vi "add to cycle cluster.vi"(6 "data requested":string[](array[string])=["q", "ratio", "norm", "error", "percent error", "delta q", "use", "break"], 7 "charge state":dbl=3.0, 8 "error in":errorcluster, 11 "input cluster":T1 {"cycle results dbl" format="%#_11f"}) -> (0 "error out":errorcluster, 3 "output cluster":T1 {"cycle results dbl" format="%#_11f"})   [LabVIEW 2016]
uses:
  controls/cycle results control.ctl
panel:
  out "cycle results dbl 2":dbl[](array[numeric])
  out "cycle results labels 3":string[](array[string])
  out "appended array":dbl[][](array[numeric]) format="%#_6f"
  out "Array":dbl[][](array[numeric])
  out "cycle results labels 2":string[](array[string])
  out "cycle results dbl":dbl[][](array[numeric])
  out "cycle results labels":string[](array[string])
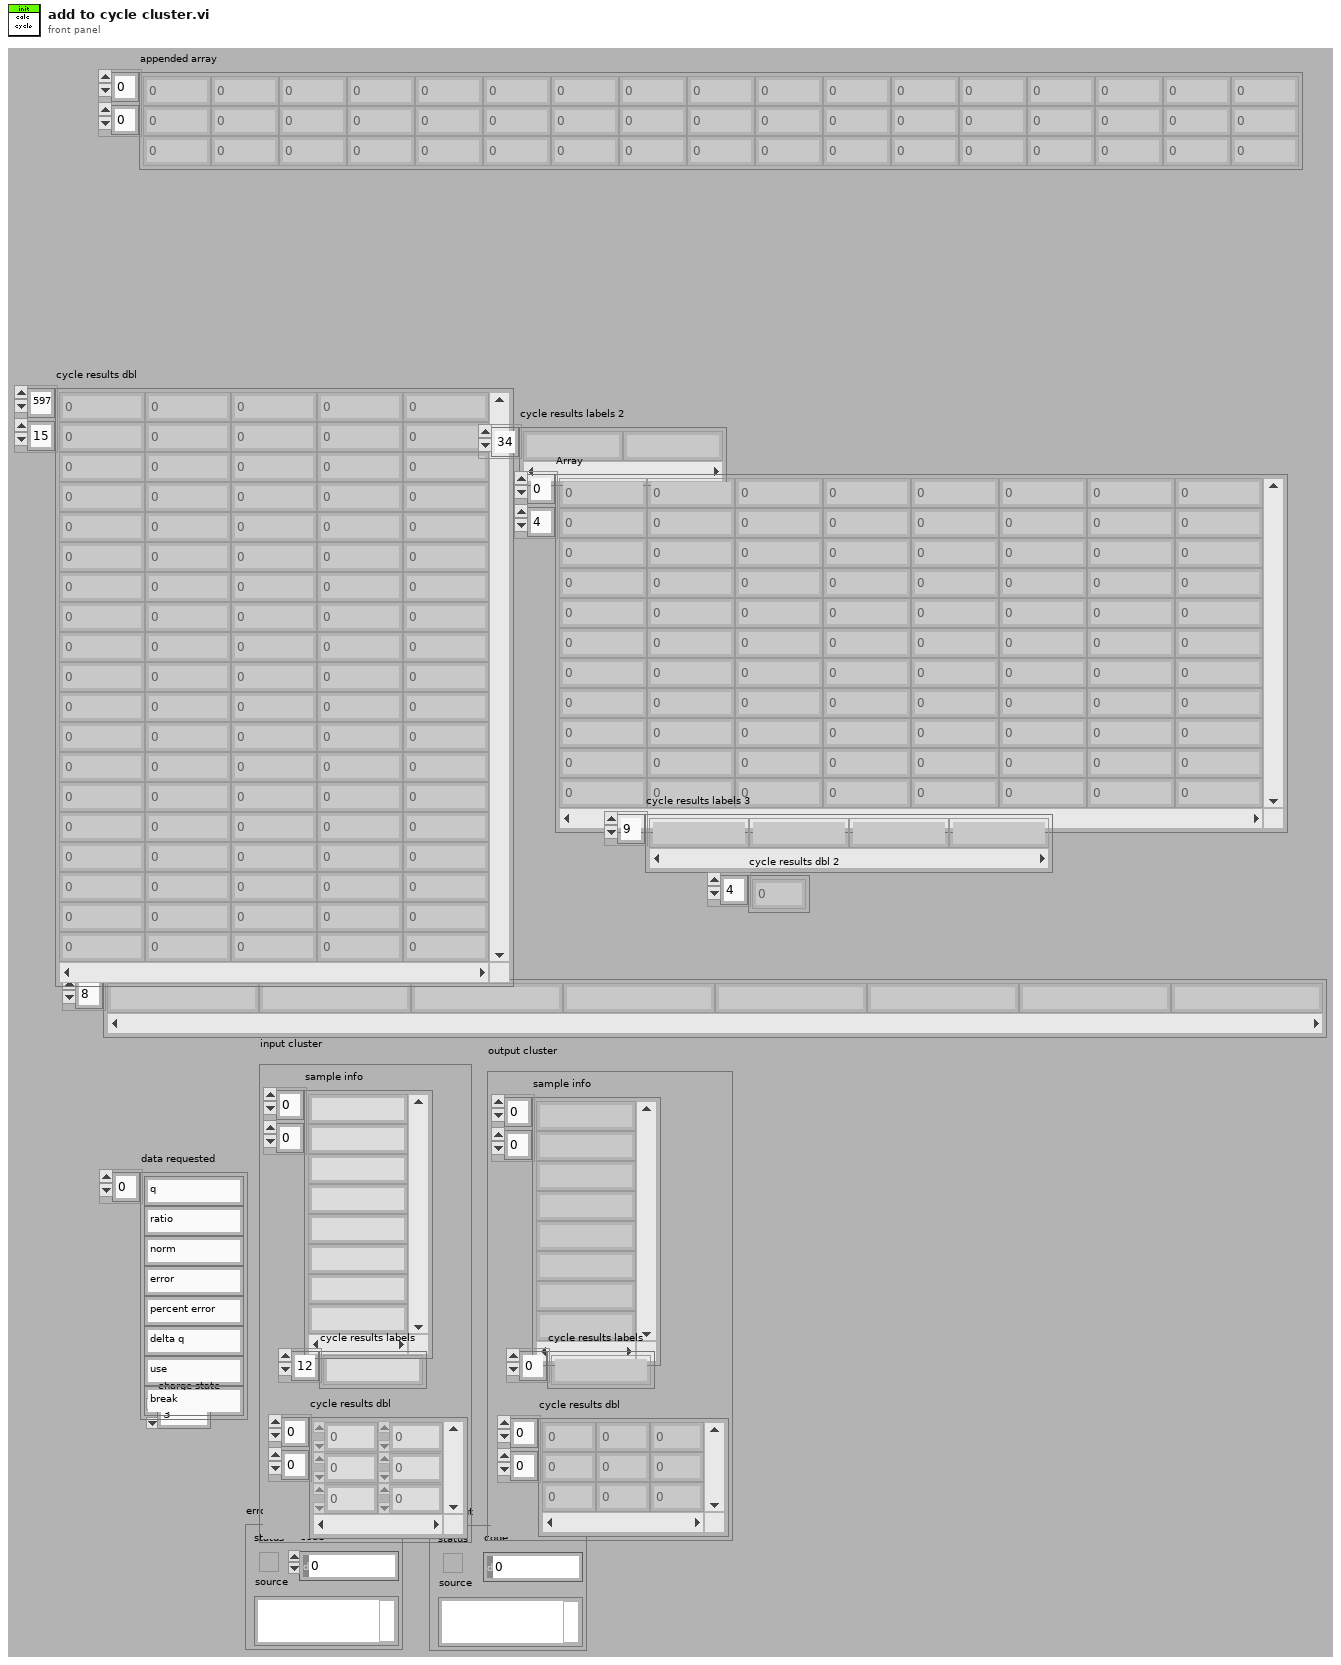
[diagram p1: front panel]
types:
  T1 = typedef "cycle results control.ctl" = cluster{"sample info":string[][], "cycle results labels":string[], "cycle results dbl":dbl[][]}
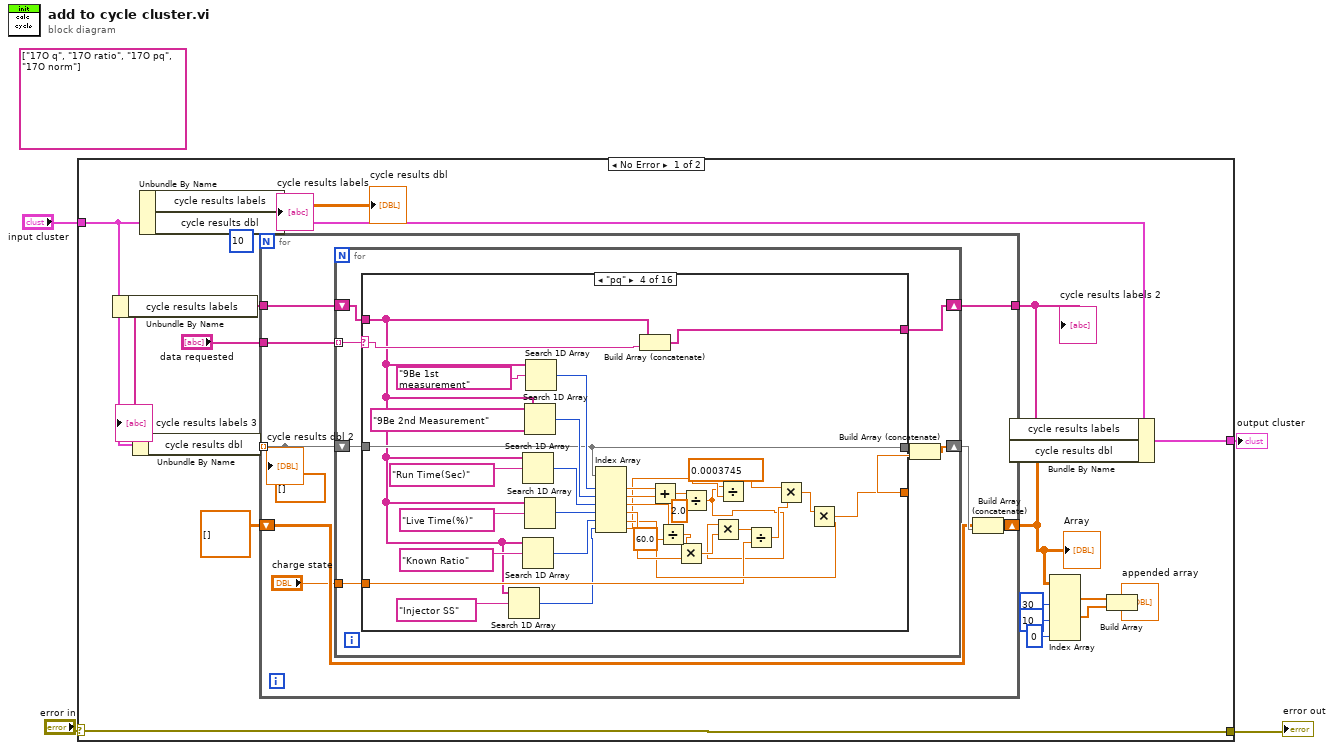
[diagram p0: block diagram]
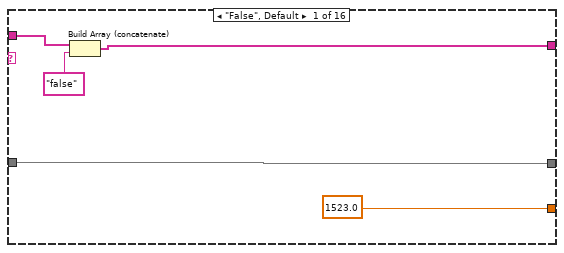
[diagram p2: hidden frame]
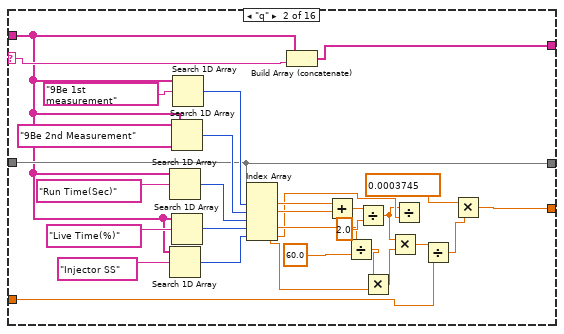
[diagram p3: hidden frame]
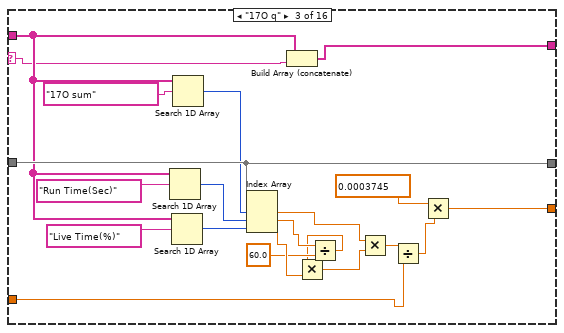
[diagram p4: hidden frame]
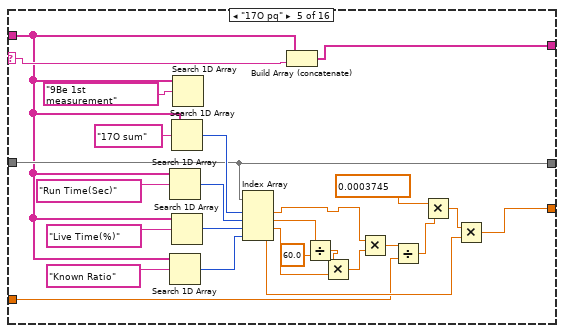
[diagram p5: hidden frame]
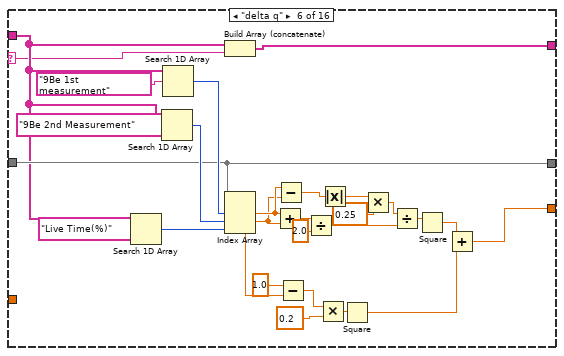
[diagram p6: hidden frame]
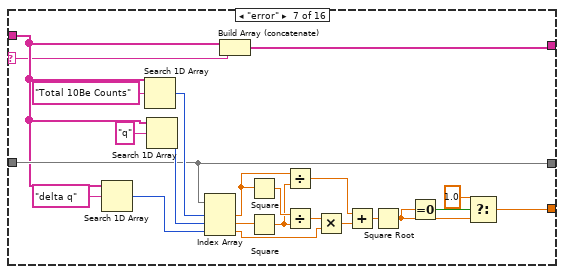
[diagram p7: hidden frame]
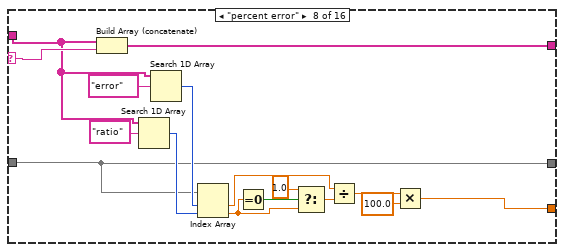
[diagram p8: hidden frame]
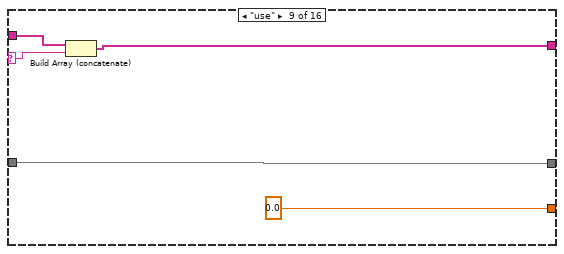
[diagram p9: hidden frame]
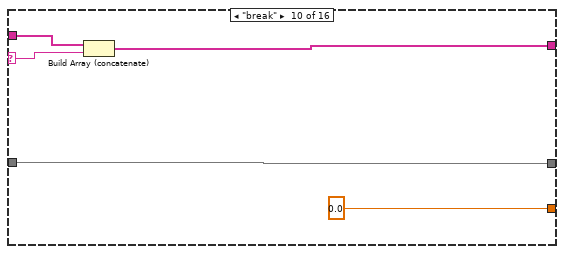
[diagram p10: hidden frame]
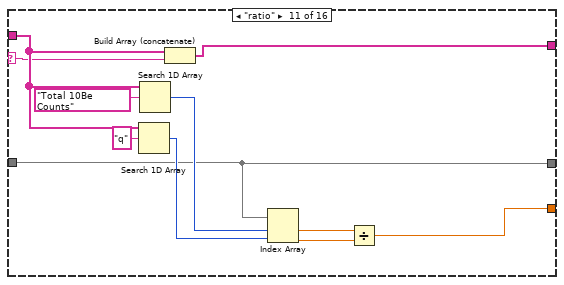
[diagram p11: hidden frame]
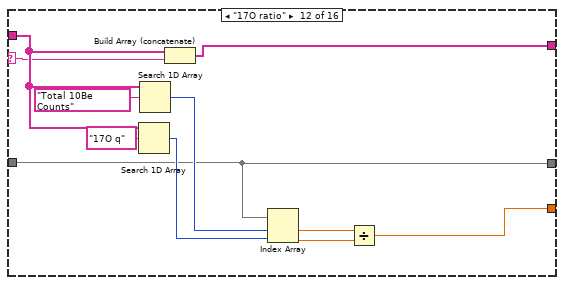
[diagram p12: hidden frame]
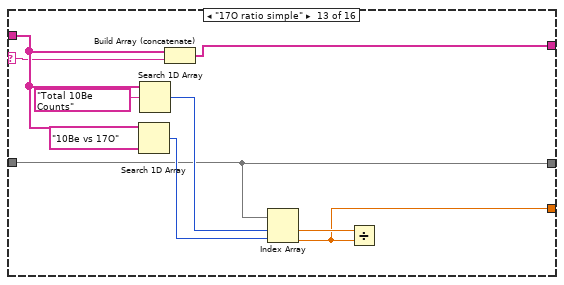
[diagram p13: hidden frame]
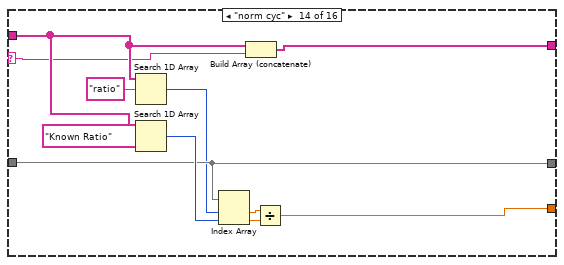
[diagram p14: hidden frame]
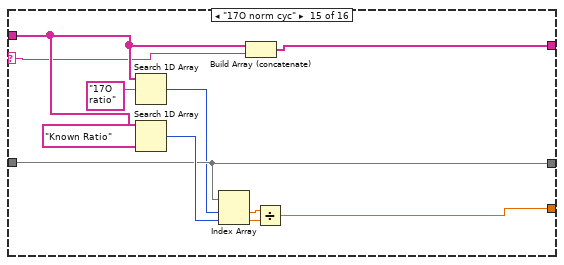
[diagram p15: hidden frame]
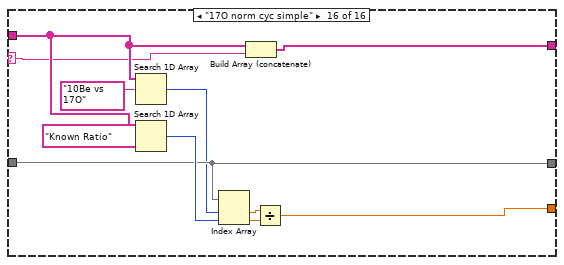
[diagram p16: hidden frame]
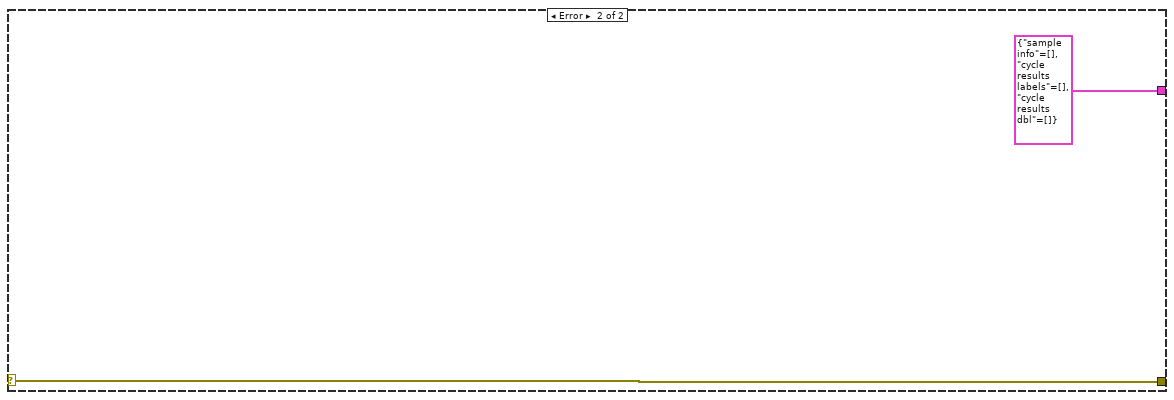
[diagram p17: hidden frame]
diagram:
  (unwired) string[] ["17O q", "17O ratio", "17O pq", "17O norm"] ("data requested")
  n1 = case shown="No Error" "error in" {
    selector: "error in" -> [w18 w297]
    tunnel: [w18 w297] -> w3
    tunnel: "input cluster" -> [w15 _]
    tunnel: [w16 T1 {"sample info"=[], "cycle results labels"=[], "cycle results dbl"=[]} ("input cluster")] -> w1
    frame No Error {
      (unwired) 10
      n2 = Unbundle By Name(w15) -> ("cycle results labels"=w17:string[])
      "cycle results labels 3" <- w17
      n3 = Unbundle By Name(w15) -> ("cycle results dbl"=w21:dbl[][])
      n4 = Unbundle By Name(w15) -> ("cycle results labels"=→"cycle results labels":string[], "cycle results dbl"=→"cycle results dbl":dbl[][])
      n5 = for {
        tunnel: w21 -> [w28] mode=indexing
        tunnel: "data requested" -> [w29]
        shift-right: [w26] -> w12
        shift-left: dbl[][] [] -> [w25]
        tunnel: [w24] -> w19
        tunnel: w17 -> [w23]
        (unwired) dbl[] []
        n6 = for {
          tunnel: w29 -> [w37] mode=indexing
          shift-right: [w34] -> w27
          shift-left: w28 -> [w33]
          shift-right: [w32] -> w24
          shift-left: w23 -> [w31]
          tunnel: "charge state" -> [w30]
          n7 = case shown="\"pq\"" w37 {
            selector: w37 -> [_ w52 w81 w107 w138 w172 w197 w215 w223 w227 w235 w246 w256 w268 w279 w290]
            tunnel: w33 -> [w41 w57 w86 w111 w142 w175 w200 w217 w224 w229 w238 w249 w259 w271 w282 w293]
            tunnel: w31 -> [w39 w49 w82 w97 w134 w173 w198 w213 w222 w228 w236 w247 w257 w269 w280 w291]
            tunnel: [1523.0 w53 w83 w100 w130 w156 w185 w210 0.0 ("t") 0.0 ("t") w231 w242 w253 w264 w275 w286] -> w36
            tunnel: [w41 w57 w86 w111 w142 w175 w200 w217 w224 w229 w238 w249 w259 w271 w282 w293] -> w35
            tunnel: [w38 w51 w80 w106 w137 w171 w196 w214 w221 w226 w234 w245 w255 w267 w278 w289] -> w32
            tunnel: w30 -> [_ w50 w78 w99 w129 _ _ _ _ _ _ _ _ _ _ _]
            frame "False", Default {
              n8 = Build Array (concatenate)(w39, "false" ("String")) -> (w38:string[])
            }
            frame "q" {
              n9 = Search 1D Array(1D array=w49, element="Run Time(Sec)") -> (index of element=w67:i32)  [unwired: 1 in]
              n10 = Search 1D Array(1D array=w49, element="Injector SS") -> (index of element=w47:i32)  [unwired: 1 in]
              n11 = Search 1D Array(1D array=w49, element="9Be 2nd Measurement") -> (index of element=w68:i32)  [unwired: 1 in]
              n12 = Search 1D Array(1D array=w49, element="Live Time(%)") -> (index of element=w60:i32)  [unwired: 1 in]
              n13 = Search 1D Array(1D array=w49, element="9Be 1st measurement") -> (index of element=w69:i32)  [unwired: 1 in]
              n14 = Index Array(array=w57, index #1=w69, index #2=w68, index #3=w67, index #4=w60, index #5=w47) -> (element #1=w65:dbl, element #2=w66:dbl, element #3=w62:dbl, element #4=w46:dbl, element #5=w45:dbl)
              n15 = Build Array (concatenate)(w49, w52) -> (w51:string[])
              n16 = Add(x=w65, y=w66) -> (x+y=w64:dbl)
              n17 = Divide(x=w62, y=60.0) -> (x/y=w44:dbl)
              n18 = Divide(x=w64, y=2.0) -> (x/y=w43:dbl)
              n19 = Multiply(x=w44, y=w46) -> (x*y=w59:dbl)
              n20 = Multiply(x=w43, y=w59) -> (x*y=w58:dbl)
              n21 = Divide(x=w43, y=w45) -> ()  [unwired: 1 out]
              n22 = Divide(x=w58, y=w50) -> (x/y=w55:dbl)
              n23 = Multiply(x=0.0003745, y=w55) -> (x*y=w53:dbl)
            }
            frame "17O q" {
              n24 = Search 1D Array(1D array=w82, element="Run Time(Sec)") -> (index of element=w90:i32)  [unwired: 1 in]
              n25 = Search 1D Array(1D array=w82, element="Live Time(%)") -> (index of element=w89:i32)  [unwired: 1 in]
              n26 = Search 1D Array(1D array=w82, element="17O sum") -> (index of element=w77:i32)  [unwired: 1 in]
              n27 = Index Array(array=w86, index #1=w77, index #2=w90, index #3=w89) -> (element #1=w76:dbl, element #2=w75:dbl, element #3=w79:dbl)
              n28 = Build Array (concatenate)(w82, w81) -> (w80:string[])
              n29 = Divide(x=w75, y=60.0) -> (x/y=w73:dbl)
              n30 = Multiply(x=w73, y=w79) -> (x*y=w88:dbl)
              n31 = Multiply(x=w76, y=w88) -> (x*y=w87:dbl)
              n32 = Divide(x=w87, y=w78) -> (x/y=w85:dbl)
              n33 = Multiply(x=0.0003745, y=w85) -> (x*y=w83:dbl)
            }
            frame "pq" {
              n34 = Search 1D Array(1D array=w97, element="Injector SS") -> (index of element=w96:i32)  [unwired: 1 in]
              n35 = Search 1D Array(1D array=w97, element="Run Time(Sec)") -> (index of element=w122:i32)  [unwired: 1 in]
              n36 = Search 1D Array(1D array=w97, element="Known Ratio") -> (index of element=w102:i32)  [unwired: 1 in]
              n37 = Search 1D Array(1D array=w97, element="9Be 2nd Measurement") -> (index of element=w123:i32)  [unwired: 1 in]
              n38 = Search 1D Array(1D array=w97, element="Live Time(%)") -> (index of element=w114:i32)  [unwired: 1 in]
              n39 = Search 1D Array(1D array=w97, element="9Be 1st measurement") -> (index of element=w124:i32)  [unwired: 1 in]
              n40 = Index Array(array=w111, index #1=w124, index #2=w123, index #3=w122, index #4=w114, index #5=w102, index #6=w96) -> (element #1=w120:dbl, element #2=w121:dbl, element #3=w117:dbl, element #4=w105:dbl, element #5=w101:dbl, element #6=w95:dbl)
              n41 = Build Array (concatenate)(w97, w107) -> (w106:string[])
              n42 = Add(x=w120, y=w121) -> (x+y=w119:dbl)
              n43 = Divide(x=w117, y=60.0) -> (x/y=w115:dbl)
              n44 = Multiply(x=w115, y=w105) -> (x*y=w113:dbl)
              n45 = Divide(x=w119, y=2.0) -> (x/y=w94:dbl)
              n46 = Multiply(x=w94, y=w113) -> (x*y=w112:dbl)
              n47 = Divide(x=w94, y=w95) -> ()  [unwired: 1 out]
              n48 = Divide(x=w112, y=w99) -> (x/y=w109:dbl)
              n49 = Multiply(x=0.0003745, y=w109) -> (x*y=w103:dbl)
              n50 = Multiply(x=w103, y=w101) -> (x*y=w100:dbl)
            }
            frame "17O pq" {
              n51 = Search 1D Array(1D array=w134, element="Run Time(Sec)") -> (index of element=w149:i32)  [unwired: 1 in]
              n52 = Search 1D Array(1D array=w134, element="Known Ratio") -> (index of element=w132:i32)  [unwired: 1 in]
              n53 = Search 1D Array(1D array=w134, element="17O sum") -> (index of element=w150:i32)  [unwired: 1 in]
              n54 = Search 1D Array(1D array=w134, element="Live Time(%)") -> (index of element=w145:i32)  [unwired: 1 in]
              n55 = Search 1D Array(1D array=w134, element="9Be 1st measurement") -> ()  [unwired: 1 in, 1 out]
              n56 = Index Array(array=w142, index #1=w150, index #2=w149, index #3=w145, index #4=w132) -> (element #1=w128:dbl, element #2=w148:dbl, element #3=w136:dbl, element #4=w131:dbl)
              n57 = Build Array (concatenate)(w134, w138) -> (w137:string[])
              n58 = Divide(x=w148, y=60.0) -> (x/y=w146:dbl)
              n59 = Multiply(x=w146, y=w136) -> (x*y=w144:dbl)
              n60 = Multiply(x=w128, y=w144) -> (x*y=w143:dbl)
              n61 = Divide(x=w143, y=w129) -> (x/y=w140:dbl)
              n62 = Multiply(x=0.0003745, y=w140) -> (x*y=w133:dbl)
              n63 = Multiply(x=w133, y=w131) -> (x*y=w130:dbl)
            }
            frame "delta q" {
              n64 = Search 1D Array(1D array=w173, element="Live Time(%)") -> (index of element=w165:i32)  [unwired: 1 in]
              n65 = Search 1D Array(1D array=w173, element="9Be 2nd Measurement") -> (index of element=w178:i32)  [unwired: 1 in]
              n66 = Search 1D Array(1D array=w173, element="9Be 1st measurement") -> (index of element=w179:i32)  [unwired: 1 in]
              n67 = Build Array (concatenate)(w173, w172) -> (w171:string[])
              n68 = Index Array(array=w175, index #1=w179, index #2=w178, index #3=w165) -> (element #1=w170:dbl, element #2=w169:dbl, element #3=w155:dbl)
              n69 = Add(x=w170, y=w169) -> (x+y=w177:dbl)
              n70 = Subtract(x=w170, y=w169) -> (x-y=w168:dbl)
              n71 = Subtract(x=1.0, y=w155) -> (x-y=w163:dbl)
              n72 = Divide(x=w177, y=2.0) -> (x/y=w160:dbl)
              n73 = Multiply(x=w163, y=0.2) -> (x*y=w158:dbl)
              n74 = Absolute Value(x=w168) -> (abs(x)=w167:dbl)
              n75 = Square(x=w158) -> (x^2=w157:dbl)
              n76 = Multiply(x=w167, y=0.25) -> (x*y=w161:dbl)
              n77 = Divide(x=w161, y=w160) -> (x/y=w159:dbl)
              n78 = Square(x=w159) -> (x^2=w154:dbl)
              n79 = Add(x=w154, y=w157) -> (x+y=w156:dbl)
            }
            frame "error" {
              n80 = Search 1D Array(1D array=w198, element="delta q") -> (index of element=w195:i32)  [unwired: 1 in]
              n81 = Search 1D Array(1D array=w198, element="Total 10Be Counts") -> (index of element=w202:i32)  [unwired: 1 in]
              n82 = Search 1D Array(1D array=w198, element="q") -> (index of element=w201:i32)  [unwired: 1 in]
              n83 = Index Array(array=w200, index #1=w202, index #2=w201, index #3=w195) -> (element #1=w193:dbl, element #2=w194:dbl, element #3=w189:dbl)
              n84 = Build Array (concatenate)(w198, w197) -> (w196:string[])
              n85 = Square(x=w193) -> (x^2=w192:dbl)
              n86 = Square(x=w194) -> (x^2=w191:dbl)
              n87 = Divide(x=w193, y=w191) -> (x/y=w184:dbl)
              n88 = Divide(x=w192, y=w191) -> (x/y=w190:dbl)
              n89 = Multiply(x=w190, y=w189) -> (x*y=w183:dbl)
              n90 = Add(x=w184, y=w183) -> (x+y=w182:dbl)
              n91 = Square Root(x=w182) -> (sqrt(x)=w186:dbl)
              n92 = Equal To 0?(x=w186) -> (x = 0?=w188:bool)
              n93 = Select(t=1.0, s=w188, f=w186) -> (s? t:f=w185:dbl)
            }
            frame "percent error" {
              n94 = Build Array (concatenate)(w213, w215) -> (w214:string[])
              n95 = Search 1D Array(1D array=w213, element="ratio") -> (index of element=w218:i32)  [unwired: 1 in]
              n96 = Search 1D Array(1D array=w213, element="error") -> (index of element=w219:i32)  [unwired: 1 in]
              n97 = Index Array(array=w217, index #1=w219, index #2=w218) -> (element #1=w207:dbl, element #2=w206:dbl)
              n98 = Equal To 0?(x=w206) -> (x = 0?=w209:bool)
              n99 = Select(t=1.0, s=w209, f=w206) -> (s? t:f=w205:dbl)
              n100 = Divide(x=w207, y=w205) -> (x/y=w212:dbl)
              n101 = Multiply(x=w212, y=100.0) -> (x*y=w210:dbl)
            }
            frame "use" {
              n102 = Build Array (concatenate)(w222, w223) -> (w221:string[])
            }
            frame "break" {
              n103 = Build Array (concatenate)(w228, w227) -> (w226:string[])
            }
            frame "ratio" {
              n104 = Search 1D Array(1D array=w236, element="q") -> (index of element=w239:i32)  [unwired: 1 in]
              n105 = Search 1D Array(1D array=w236, element="Total 10Be Counts") -> (index of element=w240:i32)  [unwired: 1 in]
              n106 = Build Array (concatenate)(w236, w235) -> (w234:string[])
              n107 = Index Array(array=w238, index #1=w240, index #2=w239) -> (element #1=w233:dbl, element #2=w232:dbl)
              n108 = Divide(x=w233, y=w232) -> (x/y=w231:dbl)
            }
            frame "17O ratio" {
              n109 = Search 1D Array(1D array=w247, element="17O q") -> (index of element=w250:i32)  [unwired: 1 in]
              n110 = Search 1D Array(1D array=w247, element="Total 10Be Counts") -> (index of element=w251:i32)  [unwired: 1 in]
              n111 = Build Array (concatenate)(w247, w246) -> (w245:string[])
              n112 = Index Array(array=w249, index #1=w251, index #2=w250) -> (element #1=w244:dbl, element #2=w243:dbl)
              n113 = Divide(x=w244, y=w243) -> (x/y=w242:dbl)
            }
            frame "17O ratio simple" {
              n114 = Search 1D Array(1D array=w257, element="10Be vs 17O") -> (index of element=w260:i32)  [unwired: 1 in]
              n115 = Search 1D Array(1D array=w257, element="Total 10Be Counts") -> (index of element=w261:i32)  [unwired: 1 in]
              n116 = Build Array (concatenate)(w257, w256) -> (w255:string[])
              n117 = Index Array(array=w259, index #1=w261, index #2=w260) -> (element #1=w254:dbl, element #2=w253:dbl)
              n118 = Divide(x=w254, y=w253) -> ()  [unwired: 1 out]
            }
            frame "norm cyc" {
              n119 = Search 1D Array(1D array=w269, element="ratio") -> (index of element=w263:i32)  [unwired: 1 in]
              n120 = Search 1D Array(1D array=w269, element="Known Ratio") -> (index of element=w272:i32)  [unwired: 1 in]
              n121 = Index Array(array=w271, index #1=w263, index #2=w272) -> (element #1=w266:dbl, element #2=w265:dbl)
              n122 = Build Array (concatenate)(w269, w268) -> (w267:string[])
              n123 = Divide(x=w266, y=w265) -> (x/y=w264:dbl)
            }
            frame "17O norm cyc" {
              n124 = Search 1D Array(1D array=w280, element="17O ratio") -> (index of element=w274:i32)  [unwired: 1 in]
              n125 = Search 1D Array(1D array=w280, element="Known Ratio") -> (index of element=w283:i32)  [unwired: 1 in]
              n126 = Index Array(array=w282, index #1=w274, index #2=w283) -> (element #1=w277:dbl, element #2=w276:dbl)
              n127 = Build Array (concatenate)(w280, w279) -> (w278:string[])
              n128 = Divide(x=w277, y=w276) -> (x/y=w275:dbl)
            }
            frame "17O norm cyc simple" {
              n129 = Search 1D Array(1D array=w291, element="10Be vs 17O") -> (index of element=w285:i32)  [unwired: 1 in]
              n130 = Search 1D Array(1D array=w291, element="Known Ratio") -> (index of element=w294:i32)  [unwired: 1 in]
              n131 = Index Array(array=w293, index #1=w285, index #2=w294) -> (element #1=w288:dbl, element #2=w287:dbl)
              n132 = Build Array (concatenate)(w291, w290) -> (w289:string[])
              n133 = Divide(x=w288, y=w287) -> (x/y=w286:dbl)
            }
          }
          n134 = Build Array (concatenate)(w35, w36) -> (w34:dbl[])
        }
        n135 = Build Array (concatenate)(w25, w27) -> (w26:dbl[][])
        "cycle results dbl 2" <- w28
      }
      "cycle results labels 2" <- w19
      "Array" <- w12
      n136 = Bundle By Name(cluster=w15, "cycle results labels"=w19, "cycle results dbl"=w12) -> (w16:T1)
      n137 = Index Array(array=w12, index (col) #1=30 ("disabled index (col)"), index (col) #2=10 ("disabled index (col)"), index (col) #3=0 ("index (col)")) -> (element #1=w9:dbl[], element #2=w8:dbl[])  [unwired: 3 in, 1 out]
      n138 = Build Array(w9, w8) -> (→"appended array":dbl[][])
    }
    frame Error {
    }
  }
  "error out" <- w3
  "output cluster" <- w1
